vi "subAcquisition_Waveform.vi"(6 "Waveform info":T3={"Waveform folder"=path "C:/Users/ZouOptics/Desktop/MATLAB codes/waveforms/12_waveforms.txt", "Movie frame rate (Hz)"=1000.0} {"Movie frame rate (Hz)" format="%0.0f"}, 7 "full path":path, 8 "error in (no error)":errorcluster, 10 "Waveform port selection":T2={"Dev2 DO lines"=["Dev2/port0/line3", "Dev2/port0/line5"], "Dev2 AO lines"=["Dev2/ao3", "Dev2/ao5"], "Patch AO line"="Dev1/ao0", "Dev1 AI lines"=["Dev1/ai0", "Dev1/ai8"], "Dev1 timing DO"="Dev1/port0/line1", "Camera timing DI"="Dev1/port0/line0", "Dev1 trigger source"="/Dev1/PFI0", "Dev2 trigger source"="/Dev2/PFI0"}, 11 "Handle in":u32) -> (0 "Error out":errorcluster, 2 "Acquisition params":T1={"Sampling rate (Hz)"=0.0, "dt (sec)"=0.0, "total time (sec)"=0.0, "# samples"=0, "Exposure time (ms)"=1000.0, "# frames"=0} {"Exposure time (ms)" format="%0.5f"; "Sampling rate (Hz)" format="%#.3f"}, 3 "Handle out":u32, 5 "AI Waveform":cluster{"xo":i32, dbl, "data":dbl[][]}(graph)={"xo"=0, 0.0001, "data"=array4x60000[240000 elements]})   [LabVIEW 2015]
panel:
  out "Camera info":cluster{"Handle in":u32, "Image file path":path}
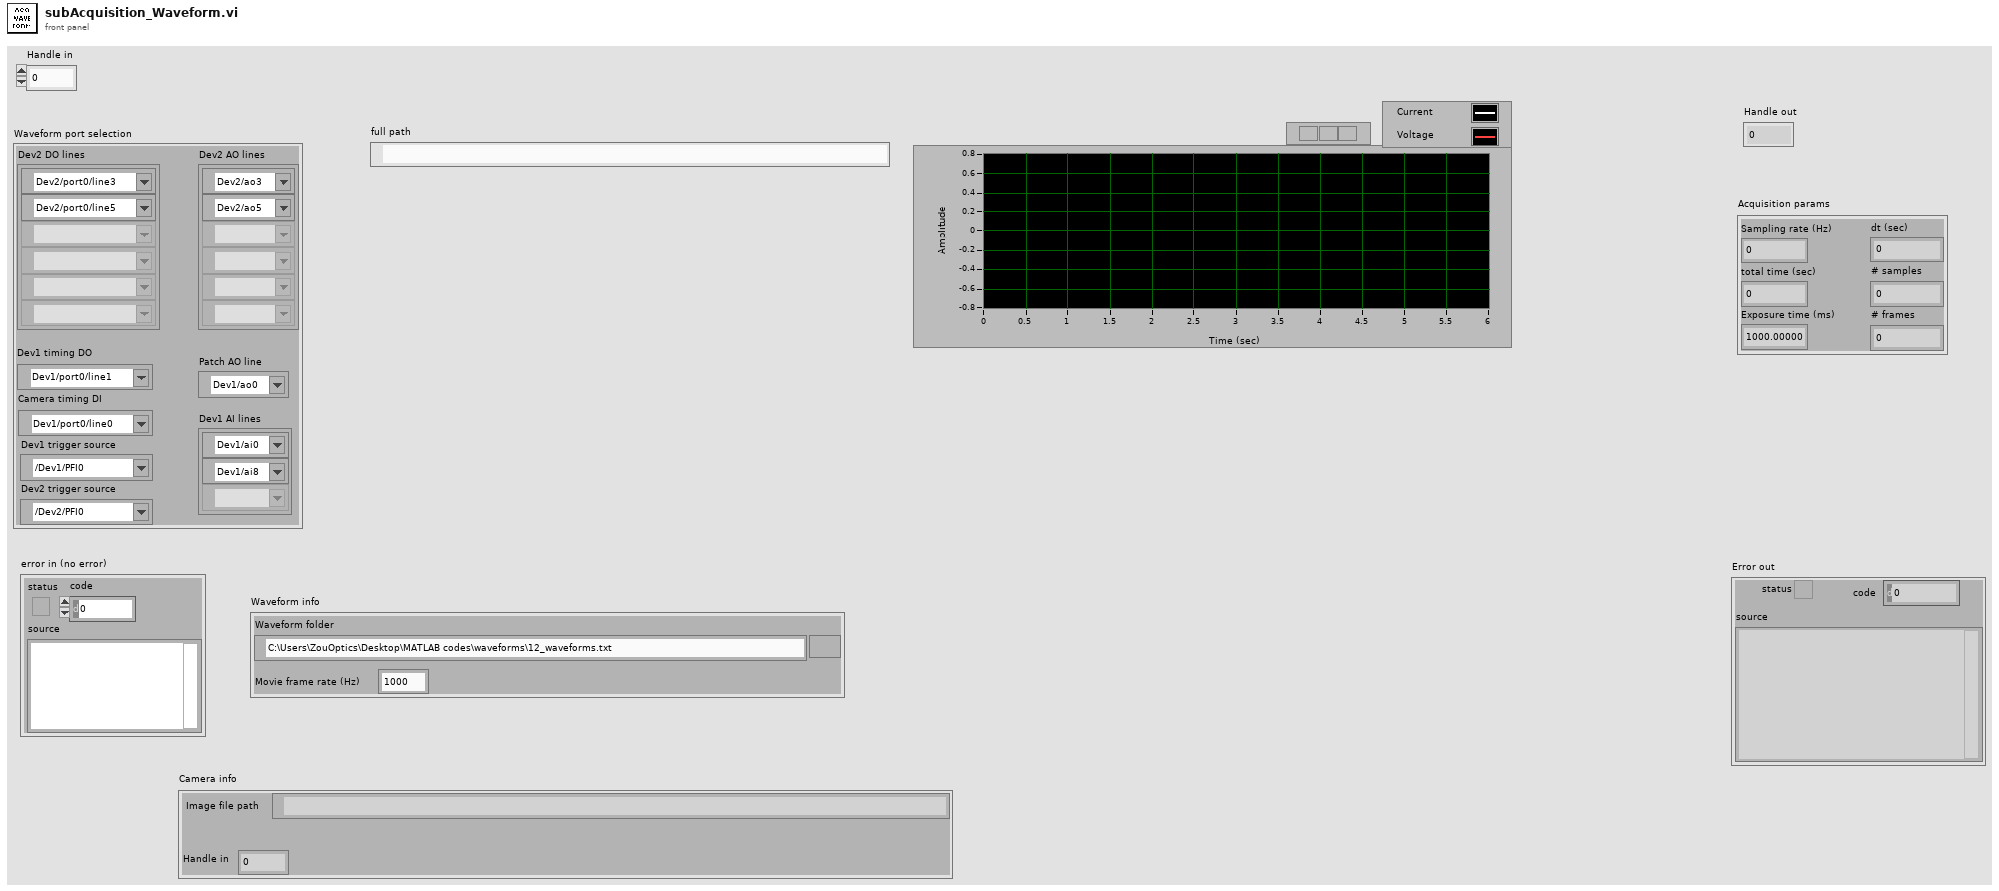
[diagram p1: front panel]
types:
  T1 = cluster{"Sampling rate (Hz)":dbl, "dt (sec)":dbl, "total time (sec)":dbl, "# samples":i32, "Exposure time (ms)":dbl, "# frames":i32}
  T2 = cluster{"Dev2 DO lines":tag[], "Dev2 AO lines":tag[], "Patch AO line":tag, "Dev1 AI lines":tag[], "Dev1 timing DO":tag, "Camera timing DI":tag, "Dev1 trigger source":tag, "Dev2 trigger source":tag}
  T3 = cluster{"Waveform folder":path, "Movie frame rate (Hz)":dbl}
  T4 = cluster{i32, "dt (sec)":dbl, "AI Waveform":dbl[][]}
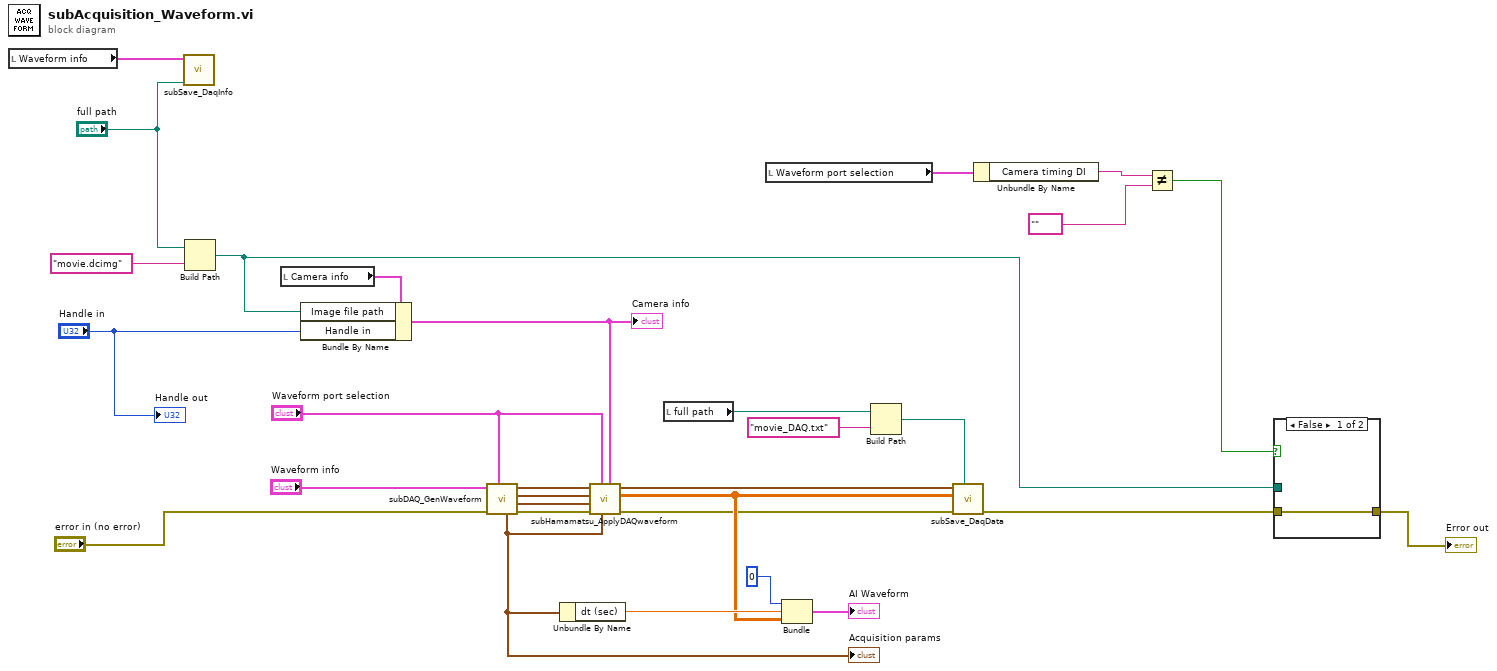
[diagram p0: block diagram]
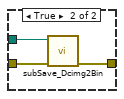
[diagram p2: hidden frame]
diagram:
  n1 = local read "Waveform info"() -> (w12:T3)
  n2 = call "subSave_DaqInfo.vi"("full path"="full path", "Waveform info"=w12) -> ()  [unwired: 10 in]
  n3 = Build Path(base path="full path", name or relative path="movie.dcimg" ("Status")) -> (appended path=w23:path)
  n4 = local read "Camera info"() -> (w22:cluster{"Handle in":u32, "Image file path":path})
  n5 = Bundle By Name(cluster=w22, "Image file path"=w23, "Handle in"="Handle in") -> (w16:cluster{"Handle in":u32, "Image file path":path})
  "Camera info" <- w16
  n6 = call "subDAQ_GenWaveform.vi"("Waveform port selection"="Waveform port selection", "error in (no error)"="error in (no error)", "Waveform info"="Waveform info") -> ("error out"=w18:errorcluster, "Dev1 AO waveform"=w19:waveform(dbl), "Lasers AO waveform"=w20:waveform(dbl)[], "Lasers DO waveform"=w21:digitalwaveform[], "Acquisition params"=w15:T1)  [unwired: 4 in]
  "Acquisition params" <- w15
  n7 = Unbundle By Name(w15) -> ("dt (sec)"=w13:dbl)
  n8 = call "subHamamatsu_ApplyDAQwaveform.vi"("Camera info"=w16, "Acquisition params"=w15, "Waveform port selection"="Waveform port selection", "Camera in (no error)"=w18, "Dev1 AO waveform"=w19, "Dev2 AO waveform"=w20, "Dev2 DO waveform"=w21) -> ("Camera out"=w6:errorcluster, "AI Waveform"=w7:dbl[][], "Camera timging DI"=w8:digitalwaveform)  [unwired: 2 in]
  n9 = local read "full path"() -> (w10:path)
  n10 = local read "Waveform port selection"() -> (w4:T2)
  n11 = Bundle(0, "dt (sec)"=w13, "AI Waveform"=w7) -> (→"AI Waveform":T4)  [unwired: 1 in]
  n12 = Build Path(base path=w10, name or relative path="movie_DAQ.txt") -> (appended path=w9:path)
  n13 = call "subSave_DaqData.vi"("path"=w9, "Camera in (no error)"=w6, "AI waveform"=w7, "DI waveform"=w8) -> ("Camera out"=w5:errorcluster)  [unwired: 7 in]
  n14 = Unbundle By Name(w4) -> ("Camera timing DI"=w3:tag)
  n15 = Not Equal?(x=w3, y=tag "") -> (x != y?=w1:bool)
  n16 = case shown="False" w1 {
    tunnel: [w31 w34] -> w25
    tunnel: w23 -> [_ w33]
    tunnel: w5 -> [w31 w32]
    frame False {
    }
    frame True {
      n17 = call "subSave_Dcimg2Bin.vi"("Error in"=w32, ".dcimg file name"=w33) -> ("Error out"=w34:errorcluster)  [unwired: 9 in]
    }
  }
  "Error out" <- w25
  "Handle out" <- "Handle in"
